vi "lv_mysql_conn_return_packet.vi"(8 "error in (no error)":errorcluster, 9 "timeout ms (5000)":i32=5000, 11 "connection ID":refnum<k5>) -> (0 "error out":errorcluster, 1 "Return Data":variant[][](array[variant]), 2 "Packet Metadata":T1 {"Server Status" format="%.0x"}, 3 "connection ID out":refnum<k5>)   [LabVIEW 2020]
uses:
  Control/ok_packet_metadata.ctl
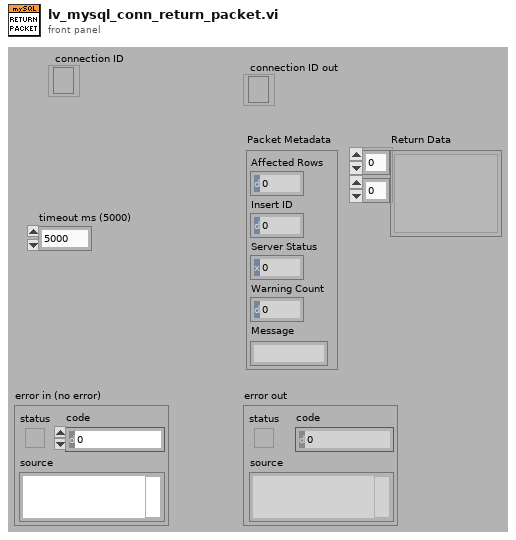
[diagram p1: front panel]
types:
  T1 = typedef "ok_packet_metadata.ctl" = cluster{"Affected Rows":u64, "Insert ID":u64, "Server Status":u16, "Warning Count":u16, "Message":string}
  T2 = typedef "return_packet_type.ctl" = enum16{"OK", "Result Set Header", "Error", "Field", "Row", "EOF"}
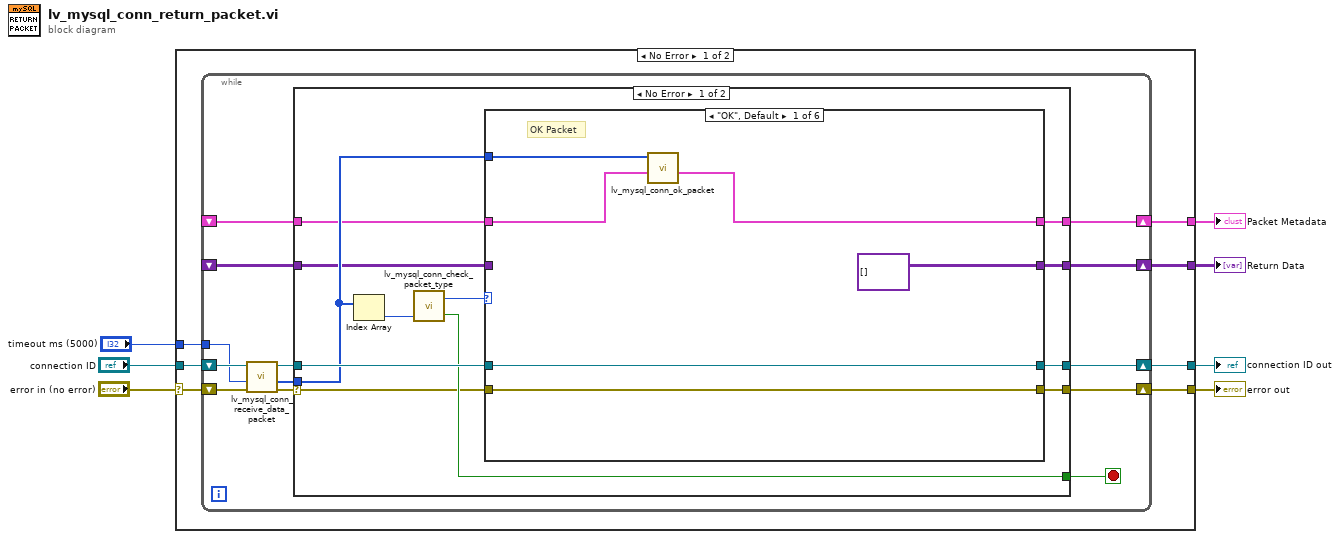
[diagram p0: block diagram]
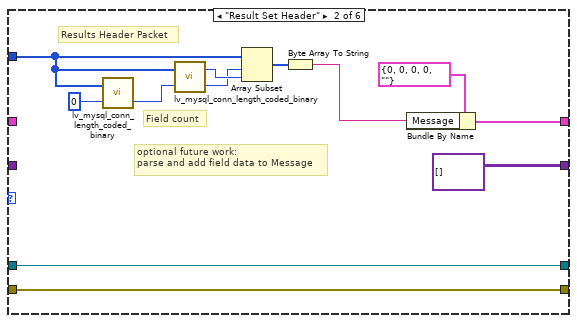
[diagram p2: hidden frame]
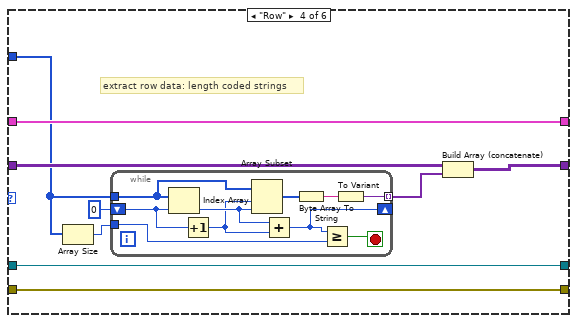
[diagram p4: hidden frame]
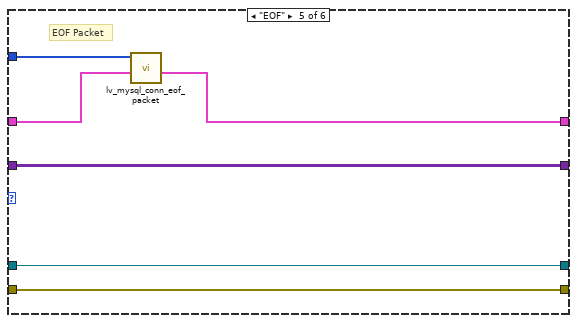
[diagram p5: hidden frame]
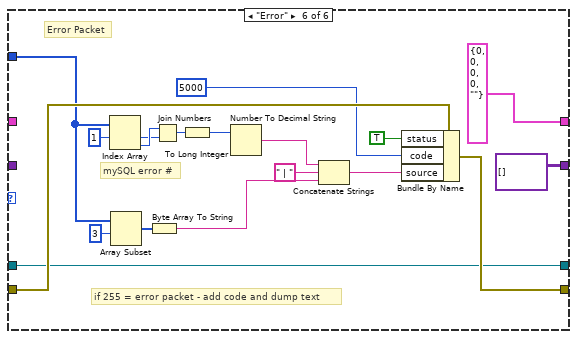
[diagram p6: hidden frame]
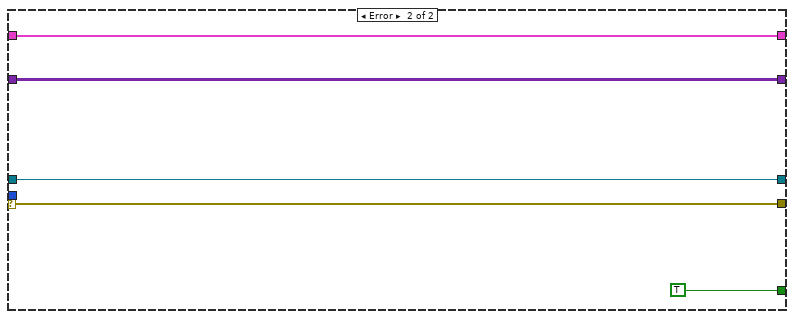
[diagram p7: hidden frame]
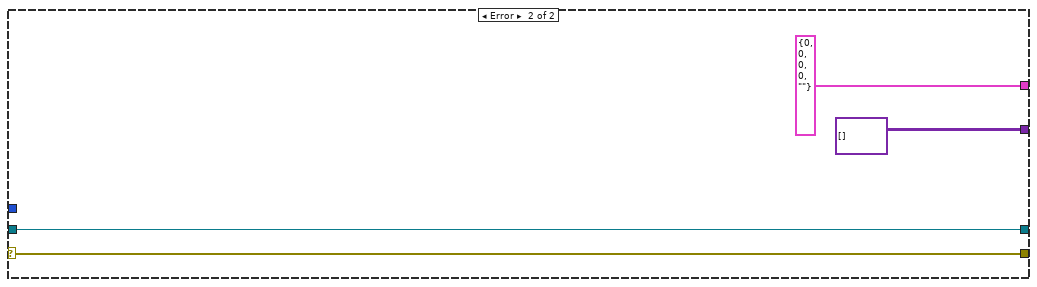
[diagram p8: hidden frame]
diagram:
  n1 = case shown="No Error" "error in (no error)" {
    selector: "error in (no error)" -> [w11 w114]
    tunnel: [w14 T1 {"Affected Rows"=0, "Insert ID"=0, "Server Status"=0, "Warning Count"=0, "Message"=""} ("OK Packet Data 2")] -> w5
    tunnel: [w12 w114] -> w7
    tunnel: [w13 variant[][] [] ("Return Data")] -> w4
    tunnel: "connection ID" -> [w10 w111]
    tunnel: [w9 w111] -> w2
    tunnel: "timeout ms (5000)" -> [w8 _]
    frame No Error {
      n2 = while {
        tunnel: w8 -> [w19]
        shift-right: [w26] -> w13
        shift-left: _ -> [w18]
        shift-right: [w25] -> w12
        shift-left: w11 -> [w24]
        shift-right: [w22] -> w9
        shift-left: w10 -> [w23]
        shift-right: [w27] -> w14
        shift-left: _ -> [w16]
        stop <- w17 stop-if-true
        n3 = call "lv_mysql_conn_receive_data_packet.vi"("error in"=w24, "timeout ms (5000)"=w19, "connection ID"=w23) -> ("error out"=w15:errorcluster, "TCP/IP Data"=w20:u8[], "connection ID out"=w21:refnum<k5>)  [unwired: 5 in, 1 out]
        n4 = case shown="No Error" w15 {
          selector: w15 -> [w30 w110]
          tunnel: [w39 w107] -> w27
          tunnel: [w38 w108] -> w26
          tunnel: [w37 w110] -> w25
          tunnel: [w36 w109] -> w22
          tunnel: w21 -> [w35 w109]
          tunnel: w20 -> [w34 _]
          tunnel: w18 -> [w29 w108]
          tunnel: [w33 TRUE ("End")] -> w17
          tunnel: w16 -> [w31 w107]
          frame No Error {
            n5 = Index Array(array=w34) -> (element=w32:u8)  [unwired: 1 in]
            n6 = call "lv_mysql_conn_check_packet_type.vi"("1st Packet Element"=w32) -> ("End"=w33:bool, "Return Packet Type"=w28:T2)  [unwired: 2 in]
            n7 = case shown="\"OK\", Default" w28 {
              tunnel: w34 -> [w45 w47 _ w63 w86 w96]
              tunnel: [w40 w56 w60 w68 w82 T1 {"Affected Rows"=0, "Insert ID"=0, "Server Status"=0, "Warning Count"=0, "Message"=""} ("OK Packet Data")] -> w39
              tunnel: [variant[][] [] ("Return Data") variant[][] [] ("Return Data") w61 w65 w81 variant[][] [] ("Return Data")] -> w38
              tunnel: w30 -> [w44 w48 w58 w69 w85 w97]
              tunnel: [w44 w48 w58 w69 w85 w95] -> w37
              tunnel: [w42 w49 w59 w70 w84 w87] -> w36
              tunnel: w35 -> [w42 w49 w59 w70 w84 w87]
              tunnel: w29 -> [_ _ w61 w66 w81 _]
              tunnel: w31 -> [w41 _ w60 w68 w83 _]
              frame "OK", Default {
                # "OK Packet"
                n8 = call "lv_mysql_conn_ok_packet.vi"("OK Packet Data In"=w41, "TCPIP Data"=w45) -> ("OK Packet Data"=w40:T1)  [unwired: 9 in]
              }
              frame "Result Set Header" {
                # "optional future work:\nparse and add field data to Message"
                # "Field count"
                # "Results Header Packet"
                n9 = call "lv_mysql_conn_length_coded_binary.vi"("Start Index"=0, "Data"=w47) -> ("Next Index"=w55:i32)  [unwired: 1 out]
                n10 = call "lv_mysql_conn_length_coded_binary.vi"("Start Index"=w55, "Data"=w47) -> ("Next Index"=w53:i32, "Output"=w54:u64)
                n11 = Array Subset(array=w47, index=w53, length=w54) -> (w52:u8[])
                n12 = Byte Array To String(unsigned byte array=w52) -> (string=w51:string)
                n13 = Bundle By Name(cluster=T1 {"Affected Rows"=0, "Insert ID"=0, "Server Status"=0, "Warning Count"=0, "Message"=""} ("OK Packet Data"), "Message"=w51) -> (w56:T1)
              }
              frame "Field" {
                # "optional future work:\nparse and add field data to metadata"
                # "Fields"
              }
              frame "Row" {
                # "extract row data: length coded strings"
                n14 = Array Size(array=w63) -> (size(s)=w62:i32)
                n15 = while {
                  tunnel: w63 -> [w79]
                  shift-right: [w72] -> _
                  shift-left: 0 -> [w78]
                  tunnel: [w80] -> w64 mode=indexing
                  tunnel: w62 -> [w71]
                  stop <- w73 stop-if-true
                  n16 = Index Array(array=w79, index=w78) -> (element=w75:u8)
                  n17 = Increment(x=w78) -> (x+1=w74:i32)
                  n18 = Array Subset(array=w79, index=w74, length=w75) -> (w77:u8[])
                  n19 = Add(x=w75, y=w74) -> (x+y=w72:i32)
                  n20 = Byte Array To String(unsigned byte array=w77) -> (string=w76:string)
                  n21 = Greater Or Equal?(x=w72, y=w71) -> (x >= y?=w73:bool)
                  n22 = To Variant(anything=w76) -> (Variant=w80:variant)
                }
                n23 = Build Array (concatenate)(w66, w64) -> (w65:variant[][])
              }
              frame "EOF" {
                # "EOF Packet"
                n24 = call "lv_mysql_conn_eof_packet.vi"("Packet Metadata In"=w83, "TCPIP Data"=w86) -> ("Packet Metadata Out"=w82:T1)  [unwired: 9 in]
              }
              frame "Error" {
                # "mySQL error #"
                # "Error Packet"
                # "if 255 = error packet - add code and dump text"
                n25 = Index Array(array=w96, index #1=1 ("index")) -> (element #1=w104:u8, element #2=w105:u8)  [unwired: 1 in]
                n26 = Array Subset(array=w96, index=3) -> (w100:u8[])  [unwired: 1 in]
                n27 = Byte Array To String(unsigned byte array=w100) -> (string=w93:string)
                n28 = Join Numbers(hi=w105, lo=w104) -> ((hi.lo)=w103:u16)
                n29 = To Long Integer(number=w103) -> (32bit integer=w90:i32)
                n30 = Number To Decimal String(number=w90) -> (decimal integer string=w89:string)  [unwired: 1 in]
                n31 = Concatenate Strings(w89, " | " ("string"), w93) -> (w92:string)
                n32 = Bundle By Name(cluster=w97, "status"=TRUE, "code"=5000, "source"=w92) -> (w95:errorcluster)
              }
            }
          }
          frame Error {
          }
        }
      }
    }
    frame Error {
    }
  }
  "error out" <- w7
  "Packet Metadata" <- w5
  "Return Data" <- w4
  "connection ID out" <- w2
